vi "mqttCmdAcknowledge.vi"(0 "mqttConnect in":refnum<class "mqttCmdConnect.lvclass">, 11 "error in (no error)":errorcluster) -> (4 "mqttConnect out":refnum<class "mqttCmdConnect.lvclass">, 8 "notification":T1, 15 "error out":errorcluster)   [LabVIEW 2017, in "mqttCmdConnect.lvclass"]
uses:
  mqttCmdConnect.lvclass
  C:/Users/mriet/Documents/VI/mqtt-LabVIEW/src/class/mqtt/mqttCmd/mqttCmd.lvclass
  mqttTypedef/mqttRXdataCluster.ctl
  mqttTypedef/mqttFixedHeaderResponse.ctl
  mqttTypedef/mqttQOSlevel.ctl
  mqttTypedef/mqttMessageType.ctl
  mqttTypedef/mqttConnectionStatus.ctl
  mqttCmdConnect.lvclass/mqttCmdConnect.ctl
  mqttCmd.lvclass/mqttCmd.ctl
  mqttCmd.lvclass
panel:
  out "payload (HEX)":u8[](array[numeric]) format="%02x"
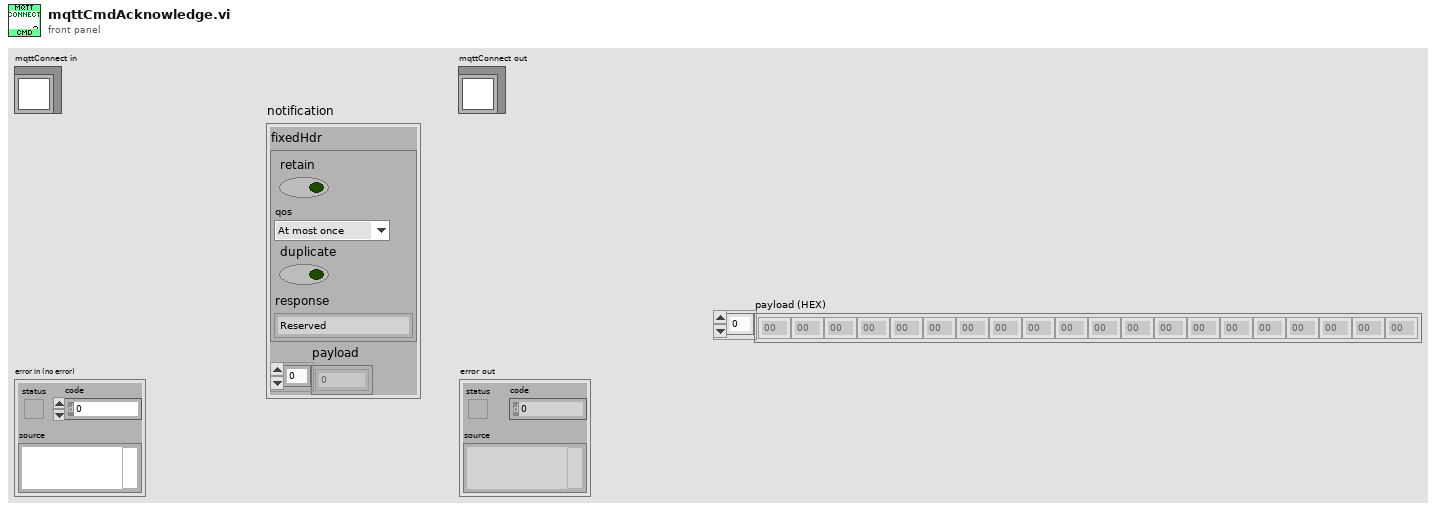
[diagram p1: front panel]
types:
  T1 = typedef "mqttRXdataCluster.ctl" = cluster{"fixedHdr":T2, "payload":u8[]}
  T2 = typedef "mqttFixedHeaderResponse.ctl" = cluster{"retain":bool, "qos":T3, "duplicate":bool, "response":T4}
  T3 = typedef "mqttQOSlevel.ctl" = enum8{"At most once", "At least once", "Exactly once", "Reserved"}
  T4 = typedef "mqttMessageType.ctl" = enum32{"Reserved", "CONNECT", "CONNACK", "PUBLISH", "PUBACK", "PUBREC", "PUBREL", "PUBCOMP", "SUBSCRIBE", "SUBACK", "UNSUBSCRIBE", "UNSUBACK", "PINGREQ", "PINGRESP", "DISCONNECT", "Reserved2"}
  T5 = typedef "mqttConnectionStatus.ctl" = enum16{"Connection accepted", "Connection refused: unacceptable protocol version", "Connection refused: identifier rejected", "Connection refused: Server unavailable", "Connection refused: bad user name or password", "Connection refused: not authorized"}
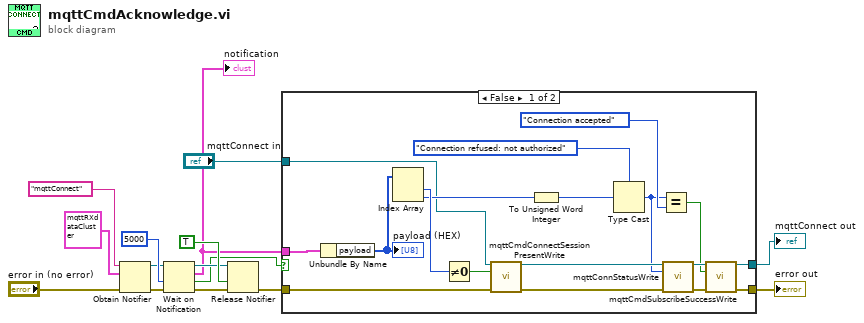
[diagram p0: block diagram]
diagram:
  n1 = Obtain Notifier(name (unnamed)="mqttConnect", notification data type=T1 {"fixedHdr"={"retain"=FALSE, "qos"=enum."At most once", "duplicate"=FALSE, "response"=enum."Reserved"}, "payload"=[]} ("output cluster"), error in (no error)="error in (no error)") -> (notifier out=w11:refnum<notifier>, error out=w10:errorcluster)  [unwired: 1 in, 1 out]
  n2 = Wait on Notification(notifier=w11, timeout in ms (-1)=5000, error in (no error)=w10) -> (notifier out=w14:refnum<notifier>, notification=w6:T1, timed out?=w1:bool, error out=w13:errorcluster)  [unwired: 1 in]
  "notification" <- w6
  n3 = Release Notifier(notifier=w14, force destroy? (F)=TRUE, error in (no error)=w13) -> (error out=w4:errorcluster)  [unwired: 2 out]
  n4 = case shown="False" w1 {
    tunnel: w6 -> [w29 _]
    tunnel: "mqttConnect in" -> [w26 w35]
    tunnel: w4 -> [w24 w34]
    tunnel: [w21 w35] -> w3
    tunnel: [w20 w34] -> w2
    frame False {
      n5 = Unbundle By Name(w29) -> ("payload"=w28:u8[])
      "payload (HEX)" <- w28
      n6 = Index Array(array=w28) -> (element #1=w33:u8, element #2=w31:u8)  [unwired: 2 in]
      n7 = Not Equal To 0?(x=w33) -> (x != 0?=w27:bool)
      n8 = call "mqttCmdConnectSessionPresentWrite.vi"("mqttConnect in"=w26, "sessionPresent"=w27, "error in (no error)"=w24) -> ("mqttConnect out"=w25:refnum<class "mqttCmdConnect.lvclass">, "error out"=w23:errorcluster)  [unwired: 11 in]
      n9 = To Unsigned Word Integer(number=w31) -> (unsigned 16bit integer=w30:u16)
      n10 = Type Cast(type=mqttConnectionStatus."Connection refused: not authorized" ("connStatus"), x=w30) -> (*(type *) &x=w17:T5)
      n11 = Equal?(x=w17, y=mqttConnectionStatus."Connection accepted") -> (x = y?=w16:bool)
      n12 = call "mqttConnStatusWrite.vi"("mqttConnect in"=w25, "connStatus"=w17, "error in (no error)"=w23) -> ("mqttConnect out"=w22:refnum<class "mqttCmdConnect.lvclass">, "error out"=w19:errorcluster)  [unwired: 11 in]
      n13 = call "mqttCmdSubscribeSuccessWrite.vi"("mqttBrokerCommand in"=w22, "success"=w16, "error in (no error)"=w19) -> ("mqttBrokerCommand out"=w21:refnum<class "mqttCmdConnect.lvclass">, "error out"=w20:errorcluster)  [unwired: 11 in]
    }
    frame True {
    }
  }
  "error out" <- w2
  "mqttConnect out" <- w3
